vi "DllFxpMulTemp.vi"(6 "ready for output":bool, 8 "input valid":bool, 9 "enable":bool, 10 "y":fxp<+/-,64,32>, 11 "x":fxp<+/-,64,32>) -> (0 "output valid":bool, 2 "overflow?":bool, 3 "z":fxp<+,1,1>, 4 "ready for input":bool)   [LabVIEW 2017]
uses:
  <vilib>/rvi/FXPMathLib/FxpMul/subVIs/nifxpmath_Mul_SimConfig.ctl
  <vilib>/fxp/LVFixedPointQuantizationPolicyTypeDef.ctl
  <vilib>/fxp/LVFixedPointOverflowPolicyTypeDef.ctl
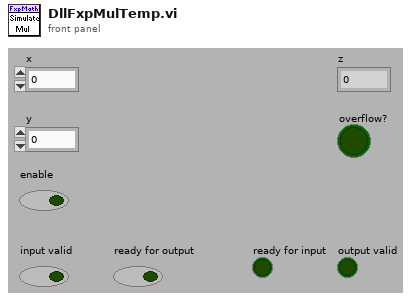
[diagram p1: front panel]
types:
  T1 = typedef "nifxpmath_Mul_SimConfig.ctl" = cluster{"kXSigned":bool, "kXWl":u32, "kXIwl":i32, "kYSigned":bool, "kYWl":u32, "kYIwl":i32, "kZSigned":bool, "kZWl":u32, "kZIwl":i32, "kNumOfStages":i32, "Fixed-Point:Quantization Policy":T2, "Fixed-Point:Overflow Policy":T3, "kSupportSCTL":bool, "kInputRegister":bool, "kOutputRegister":bool, "kShowEnable":bool}
  T2 = typedef "LVFixedPointQuantizationPolicyTypeDef.ctl" = enum32{"Truncate", "Round-Half-Up (Asymmetric)", "Round-Half-Even"}
  T3 = typedef "LVFixedPointOverflowPolicyTypeDef.ctl" = enum32{"Wrap", "Saturate"}
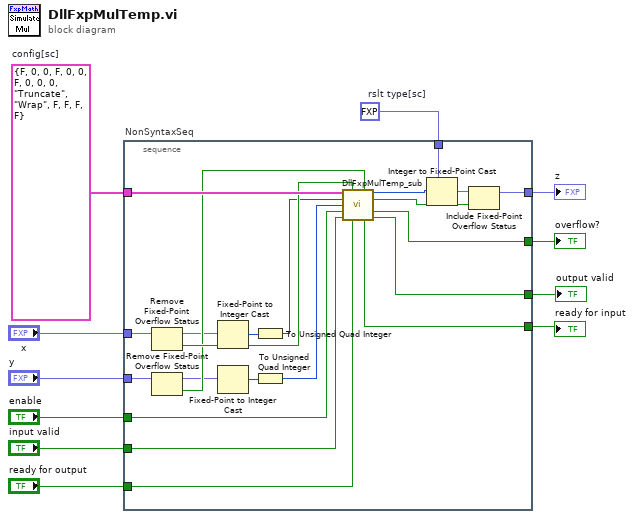
[diagram p0: block diagram]
diagram:
  w2 = T1 {"kXSigned"=FALSE, "kXWl"=0, "kXIwl"=0, "kYSigned"=FALSE, "kYWl"=0, "kYIwl"=0, "kZSigned"=FALSE, "kZWl"=0, "kZIwl"=0, "kNumOfStages"=0, "Fixed-Point:Quantization Policy"=enum."Truncate", "Fixed-Point:Overflow Policy"=enum."Wrap", "kSupportSCTL"=FALSE, "kInputRegister"=FALSE, "kOutputRegister"=FALSE, "kShowEnable"=FALSE}  # config[sc]
  w9 = fxp<+,1,1> 0.0  # rslt type[sc]
  n1 = stacked-sequence "NonSyntaxSeq" {
    tunnel: w2 -> [w31]
    tunnel: "x" -> [w33]
    tunnel: "y" -> [w32]
    tunnel: w9 -> [w12]
    tunnel: [w25] -> w8
    tunnel: "input valid" -> [w28]
    tunnel: "ready for output" -> [w27]
    tunnel: [w24] -> w5
    tunnel: [w23] -> w4
    tunnel: [w22] -> w3
    tunnel: "enable" -> [w15]
    frame #0 {
      n2 = Remove Fixed-Point Overflow Status(3:w33) -> (0:w30:bool, 1:w21:fxp<+/-,64,32>)
      n3 = Remove Fixed-Point Overflow Status(3:w32) -> (0:w29:bool, 1:w17:fxp<+/-,64,32>)
      n4 = Fixed-Point to Integer Cast(1:w21) -> (0:w20:i64)
      n5 = Fixed-Point to Integer Cast(1:w17) -> (0:w18:i64)
      n6 = To Unsigned Quad Integer(1:w20) -> (0:w19:u64)
      n7 = To Unsigned Quad Integer(1:w18) -> (0:w16:u64)
      n8 = call <vilib>:"DllFxpMulTemp_sub.vi"("config[sc]"=w31, "x ovfl status"=w30, "y ovfl status"=w29, "x"=w19, "y"=w16, "enable"=w15, "input valid"=w28, "ready for output"=w27) -> ("x*y"=w13:u64, "x*y ovfl status"=w26:bool, "overflow"=w24:bool, "ready for input"=w22:bool, "output valid"=w23:bool)  [unwired: 3 in]
      n9 = Integer to Fixed-Point Cast(fixed-point type=w12, integer=w13) -> (fixed-point=w14:fxp<+,1,1>)
      n10 = Include Fixed-Point Overflow Status(2:w26, 3:w14) -> (1:w25:fxp<+,1,1>)
    }
  }
  "overflow?" <- w5
  "z" <- w8
  "output valid" <- w4
  "ready for input" <- w3
